vi "Run.vi"(8 "error in (no error)":errorcluster, 11 "PmuAnalysis in":refnum<class "PmuAnalysis.lvclass">) -> (0 "error out":errorcluster, 2 "TimeOut":bool, 3 "PmuAnalysis out":refnum<class "PmuAnalysis.lvclass">)   [LabVIEW 2018, in "AnalysisPlugins.lvlib" / "PmuAnalysis.lvclass"]
uses:
  PmuAnalysis.lvclass
  C:/projects/ICDAS/NistPluggableModules/Analysis/AnalysisPlugins/FitterBaseClass/FitterBase.lvclass
  FitterBaseClass/FitterBase.lvclass
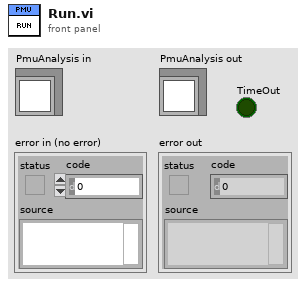
[diagram p1: front panel]
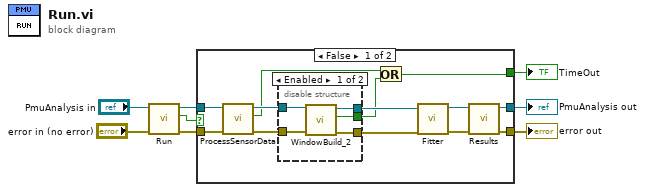
[diagram p0: block diagram]
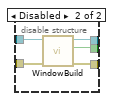
[diagram p2: hidden frame]
diagram:
  n1 = call-parent "Run.vi"("error in (no error)"="error in (no error)", "FitterBase in"="PmuAnalysis in") -> ("error out"=w6:errorcluster, "TimeOut"=w2:bool, "FitterBase out"=w5:refnum<class "PmuAnalysis.lvclass">)  [unwired: 7 in]
  n2 = case shown="False" w2 {
    selector: w2 -> [_ w32]
    tunnel: w6 -> [w17 w33]
    tunnel: w5 -> [w16 w34]
    tunnel: [w19 w34] -> w4
    tunnel: [w18 w33] -> w3
    tunnel: [w9 w32] -> w1
    frame False {
      n3 = call-dynamic "ProcessSensorData.vi"("error in (no error)"=w17, "PmuAnalysis"=w16) -> ("error out"=w15:errorcluster, "TimedOut"=w11:bool, "PMUAnalysis"=w14:refnum<class "PmuAnalysis.lvclass">)  [unwired: 7 in]
      n4 = disable-structure shown="Enabled" {
        disable-tunnel: w15 -> [w26 w31]
        disable-tunnel: w14 -> [w25 w30]
        disable-tunnel: [w24 w29] -> w13
        disable-tunnel: [w23 w27] -> w12
        disable-tunnel: [w22 w28] -> w10
        frame Enabled {
          n5 = call "WindowBuild_2.vi"("Error In"=w26, "Fitter in"=w25) -> ("Error Out"=w23:errorcluster, "Timeout"=w22:bool, "Fitter out"=w24:refnum<class "PmuAnalysis.lvclass">)  [unwired: 7 in]
        }
        frame Disabled {
          n6 = call "WindowBuild.vi"("error in (no error)"=w31, "Fitter in"=w30) -> ("error out"=w27:errorcluster, "Timeout"=w28:bool, "Fitter out"=w29:refnum<class "PmuAnalysis.lvclass">)  [unwired: 7 in]
        }
      }
      n7 = Or(x=w11, y=w10) -> (x .or. y?=w9:bool)
      n8 = call-dynamic "Fitter.vi"("error in (no error)"=w12, "PmuAnalysis in"=w13) -> ("error out"=w21:errorcluster, "PmuAnalysis out"=w20:refnum<class "PmuAnalysis.lvclass">)  [unwired: 8 in]
      n9 = call-dynamic "Results.vi"("error in (no error)"=w21, "PmuAnalysis in"=w20) -> ("error out"=w18:errorcluster, "PmuAnalysis out"=w19:refnum<class "PmuAnalysis.lvclass">)  [unwired: 8 in]
    }
    frame True {
    }
  }
  "error out" <- w3
  "PmuAnalysis out" <- w4
  "TimeOut" <- w1
